vi "Start Delay Verification.vi"(10 "Minimum sequence step dt":dbl[](array[numeric]), 11 "Start delays":dbl[](array[numeric])) -> (2 "Unsupported Start Delay?":bool[](array[boolean]), 3 "Start delays":dbl[](array[numeric]))   [LabVIEW 2024, in "devicePowerSequencerCoreLogic.lvlib"]
uses:
  devicePowerSequencerCoreLogic.lvlib
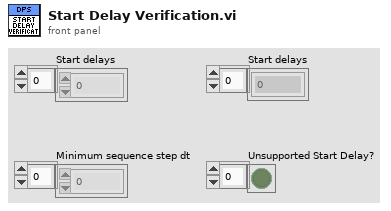
[diagram p1: front panel]
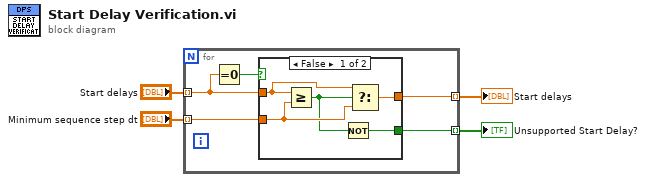
[diagram p0: block diagram]
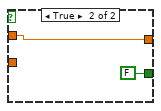
[diagram p2: hidden frame]
diagram:
  n1 = for {
    tunnel: "Start delays" -> [w6] mode=indexing
    tunnel: "Minimum sequence step dt" -> [w9] mode=indexing
    tunnel: [w8] -> w2 mode=indexing
    tunnel: [w7] -> w1 mode=indexing
    n2 = Equal To 0?(x=w6) -> (x = 0?=w5:bool)
    n3 = case shown="False" w5 {
      tunnel: w9 -> [w14 _]
      tunnel: [w13 w16] -> w8
      tunnel: [w10 FALSE] -> w7
      tunnel: w6 -> [w11 w16]
      frame False {
        n4 = Greater Or Equal?(x=w11, y=w14) -> (x >= y?=w12:bool)
        n5 = Not(x=w12) -> (.not. x?=w10:bool)
        n6 = Select(t=w11, s=w12, f=w14) -> (s? t:f=w13:dbl)
      }
      frame True {
      }
    }
  }
  "Start delays" <- w2
  "Unsupported Start Delay?" <- w1
